vi "Launch Cap Bank Server.vi"() -> ()   [LabVIEW 2015]
uses:
  Libraries/Mag Lab Measure/Mag Lab Measure Controller/Mag Lab Measure Controller.lvclass
  Libraries/Mag Lab Measure/Mag Lab Measure Controller/Cap Bank Server/Load App.vi
panel:
  out "Current action:":string
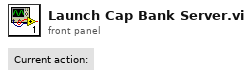
[diagram p1: front panel]
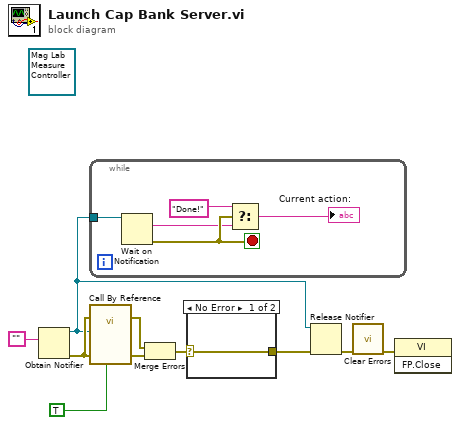
[diagram p0: block diagram]
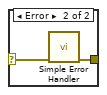
[diagram p2: hidden frame]
diagram:
  (unwired) refnum<class "Mag Lab Measure Controller.lvclass"> refnum ("Mag Lab Measure Controller.lvclass")
  n1 = Obtain Notifier(notification data type="") -> (notifier out=w2:refnum<notifier>, error out=w9:errorcluster)  [unwired: 3 in, 1 out]
  n2 = while {
    tunnel: w2 -> [w15]
    stop <- w14 stop-if-true
    n3 = Wait on Notification(notifier=w15) -> (notification=w12:string, error out=w14:errorcluster)  [unwired: 3 in, 2 out]
    n4 = Select(t="Done!" ("notification"), s=w14, f=w12) -> (s? t:f=→"Current action:":string)
  }
  n5 = call-by-ref "?"(error in=w9, "Open Actor Core front panel? (F)"=TRUE, "Error In"=w9, "Status Notifier"=w2) -> (error out=w6:errorcluster, "Error Out"=w7:errorcluster)  [unwired: 9 in, 1 out]
  n6 = Merge Errors(w6, w7) -> (w5:errorcluster)
  n7 = case shown="No Error" w5 {
    selector: w5 -> [w16 w18]
    tunnel: [w16 w17] -> w4
    frame No Error {
    }
    frame Error {
      n8 = call <vilib>:"Simple Error Handler.vi"("error in (no error)"=w18) -> ("error out"=w17:errorcluster)  [unwired: 4 in, 4 out]
    }
  }
  n9 = Release Notifier(notifier=w2, error in (no error)=w4) -> (error out=w8:errorcluster)  [unwired: 1 in, 2 out]
  n10 = call <vilib>:"Clear Errors.vi"("error in (no error)"=w8) -> ("error out"=w3:errorcluster)  [unwired: 5 in, 1 out]
  n11 = invoke class="VI" method="FP.Close"(error in=w3) -> ()  [unwired: 2 in, 3 out]
